vi "Execute Turn.vi"(7 "Player Color":T1, 8 "error in":errorcluster, 9 "Possible Moves":bool[][](array[boolean]), 10 "Board":T3[][](array[typedef]), 11 "Human in":refnum<class "Human.lvclass">) -> (0 "error out":errorcluster, 2 "Choice Coordinates":T2, 3 "Human out":refnum<class "Human.lvclass">)   [LabVIEW 2020, in "Reversi.lvlib" / "Human.lvclass"]
uses:
  Human.lvclass
  Space Ring.ctl
  Space Coordinates.ctl
  Turn Enum.ctl
  Human.lvclass/Human.ctl
  Reversi.lvclass
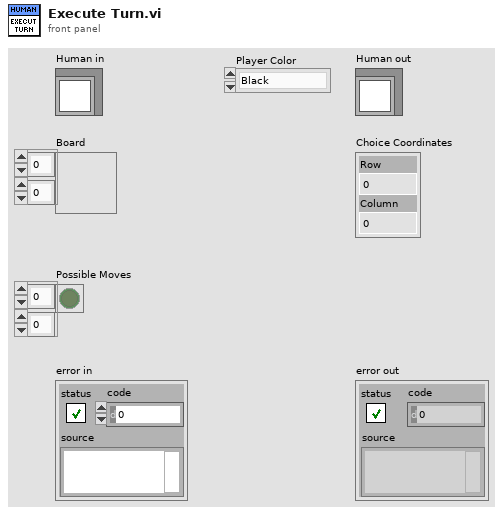
[diagram p1: front panel]
types:
  T1 = typedef "Reversi.lvlib/Reversi.lvclass/Turn Enum.ctl" = enum16{"Black", "White"}
  T2 = typedef "Reversi.lvlib/Reversi.lvclass/Space Coordinates.ctl" = cluster{"Row":i32, "Column":i32}
  T3 = typedef "Reversi.lvlib/Reversi.lvclass/Space Ring.ctl" = u16
  T4 = typedef "LVPoint32TypeDef.ctl" = cluster{"Horizontal":i32, "Vertical":i32}
  T5 = typedef "LVPositionTypeDef.ctl" = cluster{"Left":i32, "Top":i32}
  T6 = typedef "LVBoundsTypeDef.ctl" = cluster{"Width":u32, "Height":u32}
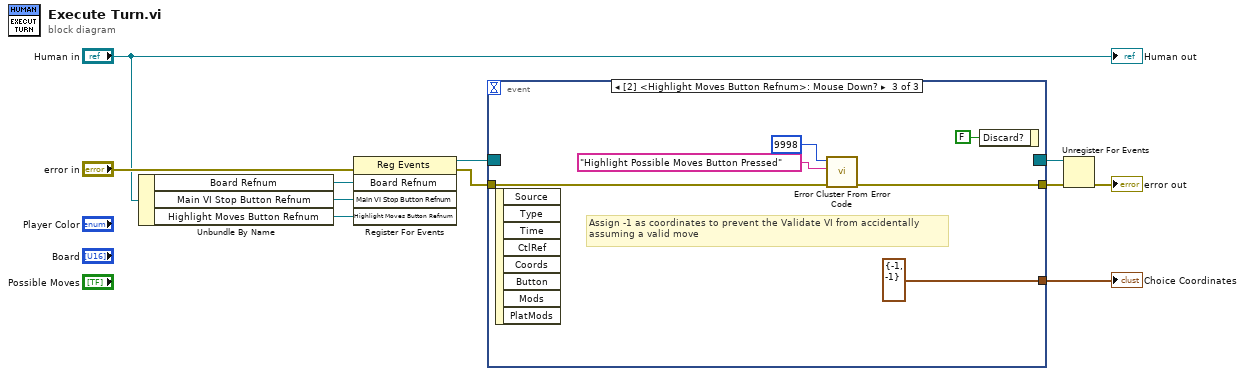
[diagram p0: block diagram]
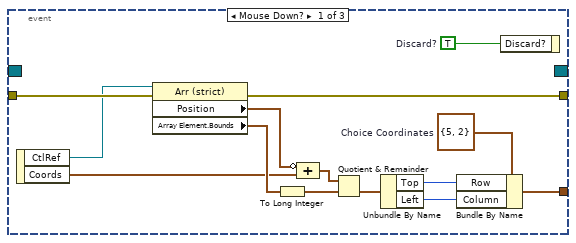
[diagram p2: hidden frame]
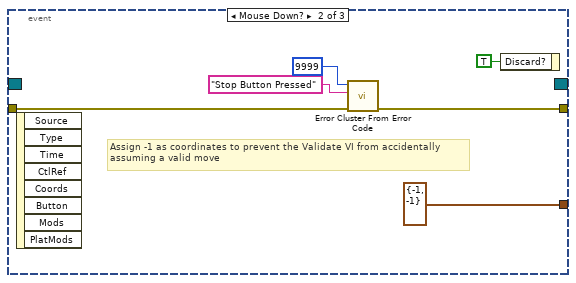
[diagram p3: hidden frame]
diagram:
  n1 = Unbundle By Name("Human in") -> ("Board Refnum"=w6:refnum<vi>, "Main VI Stop Button Refnum"=w2:refnum<vi>, "Highlight Moves Button Refnum"=w1:refnum<vi>)
  n2 = register-events(error in="error in", w6, w2, w1) -> (reference out=w5:refnum<event-registration>, error out=w10:errorcluster)  [unwired: 1 in]
  n3 = event shown="[2] <Highlight Moves Button Refnum>: Mouse Down?" {
    selector: w5 -> [_ _ _]
    dyn-events: [_ _ _] -> w3
    timeout: _ -> [_ _ _]
    tunnel: w10 -> [w25 w30 w36]
    tunnel: [w15 T2 {"Row"=-1, "Column"=-1} ("Choice Coordinates") T2 {"Row"=-1, "Column"=-1} ("Choice Coordinates")] -> w4
    tunnel: [w24 w31 w37] -> w9
    event Mouse Down? {
      w16 = T2 {"Row"=5, "Column"=2}  # Choice Coordinates
      w23 = TRUE  # Discard?
      n4 = event-data() -> ("CtlRef"=w22:refnum<vi>, "Coords"=w20:T4)  [unwired: 1 in]
      n5 = property class="Arr (strict)"(reference=w22, error in=w25) -> (error out=w24:errorcluster, "Position"=w19:T5, "Array Element.Bounds"=w21:T6)  [unwired: 1 out]
      n6 = To Long Integer(number=w21) -> (32bit integer=w17:cluster{"Width":i32, "Height":i32})
      n7 = Compound Arithmetic op=ADD(invert w19, w20) -> (w18:T5)
      n8 = Quotient & Remainder(x=w18, y=w17) -> (floor(x/y)=w14:T5)  [unwired: 1 out]
      n9 = Unbundle By Name(w14) -> ("Top"=w13:i32, "Left"=w12:i32)
      n10 = Bundle By Name(cluster=w16, "Row"=w13, "Column"=w12) -> (w15:T2)
      n11 = event-data("Discard?"=w23) -> ()  [unwired: 1 in, 1 out]
    }
    event Mouse Down? {
      # "Assign -1 as coordinates to prevent the Validate VI from accidentally\nassuming a valid move"
      n12 = event-data() -> ()  [unwired: 1 in, 8 out]
      n13 = call <vilib>:"Error Cluster From Error Code.vi"("error in (no error)"=w30, "error message (\"\")"="Stop Button Pressed" ("error message (\"\")"), "error code (0)"=9999) -> ("error out"=w31:errorcluster)  [unwired: 6 in]
      n14 = event-data("Discard?"=TRUE) -> ()  [unwired: 1 in, 1 out]
    }
    event Mouse Down? {
      # "Assign -1 as coordinates to prevent the Validate VI from accidentally\nassuming a valid move"
      n15 = event-data() -> ()  [unwired: 1 in, 8 out]
      n16 = call <vilib>:"Error Cluster From Error Code.vi"("error in (no error)"=w36, "error message (\"\")"="Highlight Possible Moves Button Pressed" ("error message (\"\")"), "error code (0)"=9998) -> ("error out"=w37:errorcluster)  [unwired: 6 in]
      n17 = event-data("Discard?"=FALSE) -> ()  [unwired: 1 in, 1 out]
    }
  }
  "Choice Coordinates" <- w4
  n18 = Unregister For Events(event registration refnum=w3, error in=w9) -> (error out=→"error out":errorcluster)
  "Human out" <- "Human in"
